vi "update std eng cluster.vi"(11 "Engine Configuration in":T10) -> (3 "Engine Configuration out":T1)   [LabVIEW 2013, in "Standard Engine Configuration.lvclass"]
uses:
  Standard Engine Configuration.lvclass
  Engine Configuration.ctl
  Loop Info.ctl
  Supported Timing Sources.ctl
  Module Specific Configuration.ctl
  Module Decimation.ctl
  Module Error Configuration.ctl
  Error Actions By Category.ctl
  <vilib>/NI/Tag Bus Module Framework/runtime/error classification.ctl
  Error Actions.ctl
  <vilib>/NI/Tag Bus Module Framework/runtime/TBM module execution interface.lvclass
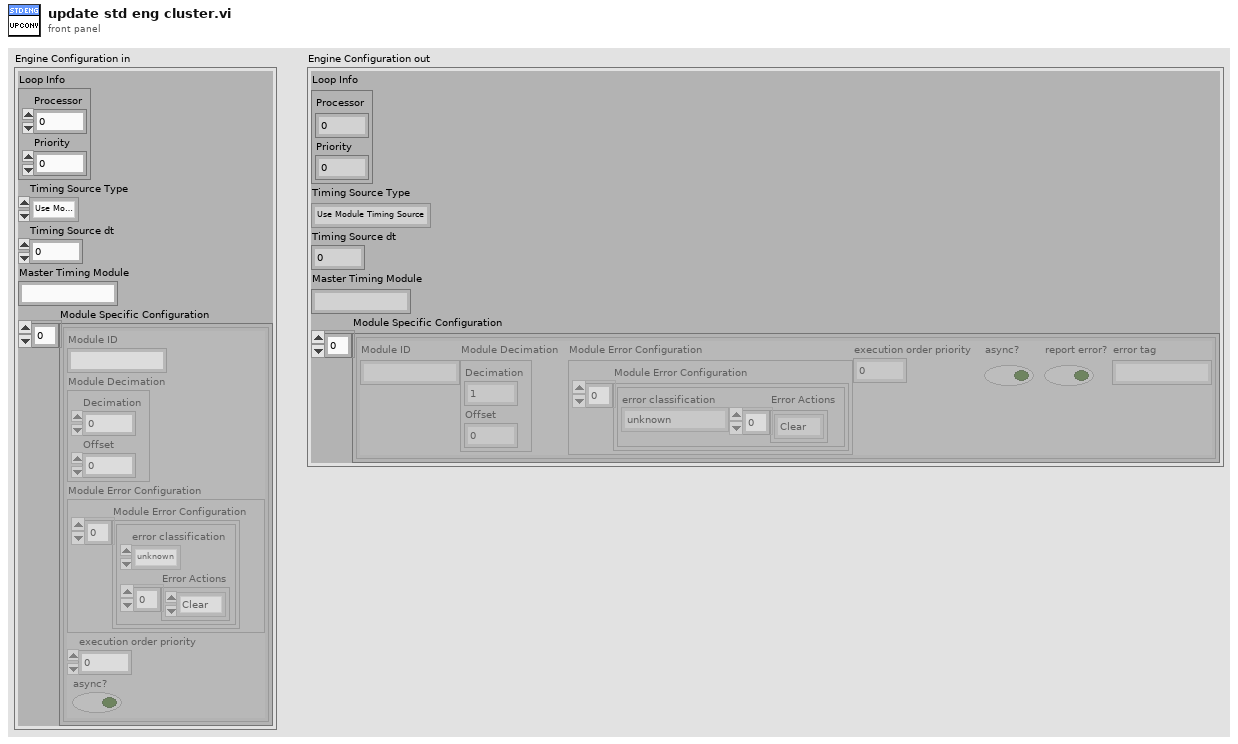
[diagram p1: front panel]
types:
  T1 = typedef "Standard Engine Configuration.lvclass/Engine Configuration.ctl" = cluster{"Loop Info":T2, "Timing Source Type":T3, "Timing Source dt":u32, "Master Timing Module":string, "Module Specific Configuration":T4[]}
  T2 = typedef "Standard Engine Configuration.lvclass/Loop Info.ctl" = cluster{"Processor":i32, "Priority":i32}
  T3 = typedef "Standard Engine Configuration.lvclass/Supported Timing Sources.ctl" = enum16{"Use Module Timing Source", "1 kHz Clock", "1 MHz Clock", "Synchronize to Scan Engine"}
  T4 = typedef "Standard Engine Configuration.lvclass/Module Specific Configuration.ctl" = cluster{"Module ID":string, "Module Decimation":T5, "Module Error Configuration":T6, "execution order priority":i32, "async?":bool, "report error?":bool, "error tag":string}
  T5 = typedef "Standard Engine Configuration.lvclass/Module Decimation.ctl" = cluster{"Decimation":u16, "Offset":u16}
  T6 = typedef "Standard Engine Configuration.lvclass/Module Error Configuration.ctl" = cluster{"Module Error Configuration":T7[]}
  T7 = typedef "Standard Engine Configuration.lvclass/Error Actions By Category.ctl" = cluster{"error classification":T8, "Error Actions":T9[]}
  T8 = typedef "TBM module execution interface.lvclass/error classification.ctl" = enum16{"unknown", "none", "trivial", "recoverable", "critical"}
  T9 = typedef "Standard Engine Configuration.lvclass/Error Actions.ctl" = enum16{"Clear", "Notify", "Stop Component", "Stop Engine", "Safe State", "Attempt Recovery"}
  T10 = cluster{"Loop Info":cluster{"Processor":i32, "Priority":i32}, "Timing Source Type":enum16{"Use Module Timing Source", "1 kHz Clock", "1 MHz Clock", "Synchronize to Scan Engine"}, "Timing Source dt":u32, "Master Timing Module":string, "Module Specific Configuration":cluster{"Module ID":string, "Module Decimation":cluster{"Decimation":u16, "Offset":u16}, "Module Error Configuration":cluster{"Module Error Configuration":cluster{"error classification":enum16{"unknown", "none", "trivial", "recoverable", "critical"}, "Error Actions":enum16{"Clear", "Notify", "Stop Component", "Stop Engine", "Safe State", "Attempt Recovery"}[]}[]}, "execution order priority":i32, "async?":bool}[]}
  T11 = enum16{"Use Module Timing Source", "1 kHz Clock", "1 MHz Clock", "Synchronize to Scan Engine"}
  T12 = cluster{"Module ID":string, "Module Decimation":cluster{"Decimation":u16, "Offset":u16}, "Module Error Configuration":cluster{"Module Error Configuration":cluster{"error classification":enum16{"unknown", "none", "trivial", "recoverable", "critical"}, "Error Actions":enum16{"Clear", "Notify", "Stop Component", "Stop Engine", "Safe State", "Attempt Recovery"}[]}[]}, "execution order priority":i32, "async?":bool}[]
  T13 = cluster{"Module Error Configuration":cluster{"error classification":enum16{"unknown", "none", "trivial", "recoverable", "critical"}, "Error Actions":enum16{"Clear", "Notify", "Stop Component", "Stop Engine", "Safe State", "Attempt Recovery"}[]}[]}
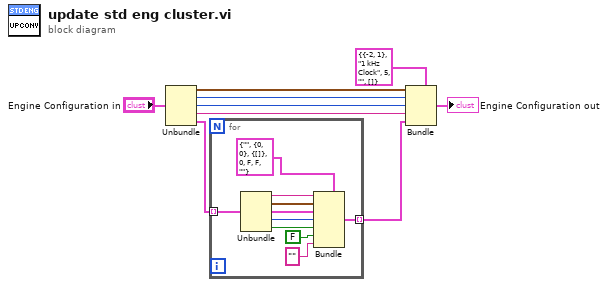
[diagram p0: block diagram]
diagram:
  n1 = Unbundle("Engine Configuration in") -> ("Loop Info"=w4:cluster{"Processor":i32, "Priority":i32}, "Timing Source Type"=w3:T11, "Timing Source dt"=w2:u32, "Master Timing Module"=w1:string, "Module Specific Configuration"=w6:T12)
  n2 = for {
    tunnel: w6 -> [w19] mode=indexing
    tunnel: [w17] -> w5 mode=indexing
    n3 = Unbundle(w19) -> ("Module ID"=w16:string, "Module Decimation"=w15:cluster{"Decimation":u16, "Offset":u16}, "Module Error Configuration"=w14:T13, "execution order priority"=w13:i32, "async?"=w12:bool)
    n4 = Bundle(cluster=T4 {"Module ID"="", "Module Decimation"={"Decimation"=0, "Offset"=0}, "Module Error Configuration"={"Module Error Configuration"=[]}, "execution order priority"=0, "async?"=FALSE, "report error?"=FALSE, "error tag"=""} ("Module Specific Configuration"), "Module ID"=w16, "Module Decimation"=w15, "Module Error Configuration"=w14, "execution order priority"=w13, "async?"=w12, "report error?"=FALSE, "error tag"="") -> (w17:T4)
  }
  n5 = Bundle(cluster=T1 {"Loop Info"={"Processor"=-2, "Priority"=1}, "Timing Source Type"=enum."1 kHz Clock", "Timing Source dt"=5, "Master Timing Module"="", "Module Specific Configuration"=[]} ("Engine Configuration"), "Loop Info"=w4, "Timing Source Type"=w3, "Timing Source dt"=w2, "Master Timing Module"=w1, "Module Specific Configuration"=w5) -> (→"Engine Configuration out":T1)
